vi "FL_SG_Filter_2.vi"(2 "SG coefficients":T1, 3 "Point of interest (can be used for extrapolation)":i32, 4 "Input array of data":dbl[](array[numeric])) -> (1 "Filtered data, 0 order":dbl)   [LabVIEW 2016]
doc: "This VI makes a Savitzky-Golay filtered of input data, length of the fitler is 31 sample, 3rd order polynom. First (and possibly last, depend on filter work mode) 15 values entered into filter will be filtered via simplified Klaman with K=0.3 instead."
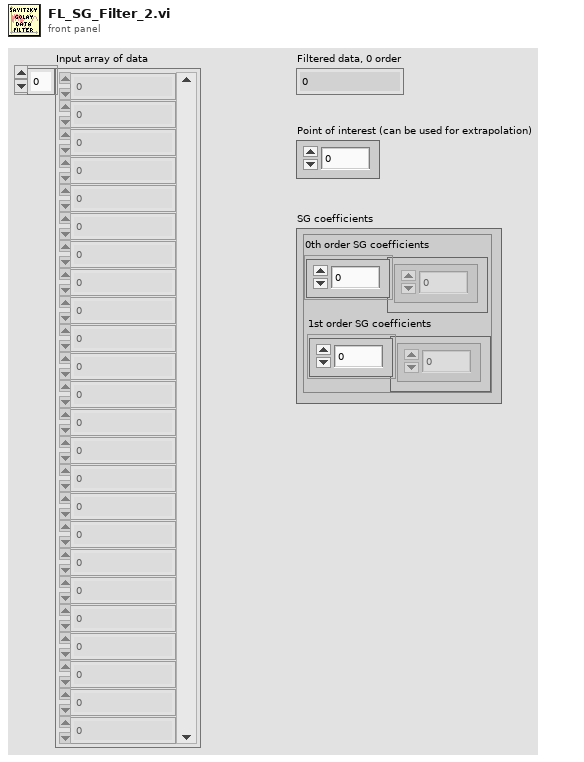
[diagram p1: front panel]
types:
  T1 = cluster{"0th order SG coefficients":dbl[], "1st order SG coefficients":dbl[]}
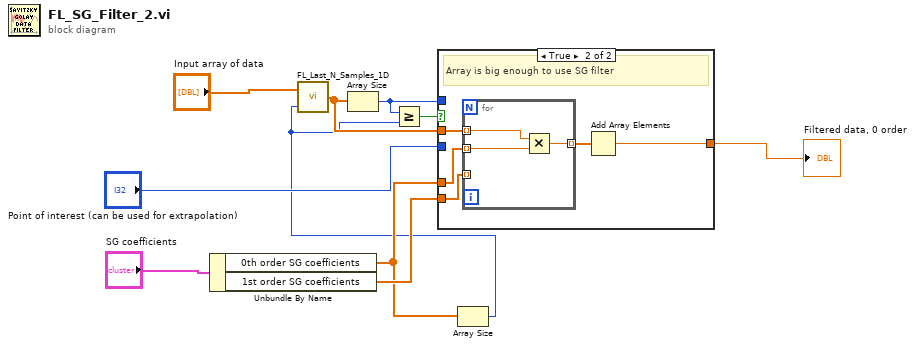
[diagram p0: block diagram]
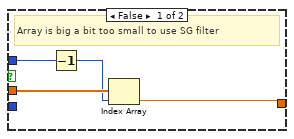
[diagram p2: hidden frame]
diagram:
  n1 = Unbundle By Name("SG coefficients") -> ("0th order SG coefficients"=w2:dbl[], "1st order SG coefficients"=w3:dbl[])
  n2 = Array Size(array=w2) -> (size(s)=w1:i32)
  n3 = call "FL_Last_N_Samples_1D.vi"("BufferLengthSamples"=w1, "Input Array of strings"="Input array of data") -> ("Output Array of strings"=w9:dbl[])
  n4 = Array Size(array=w9) -> (size(s)=w5:i32)
  n5 = Greater Or Equal?(x=w5, y=w1) -> (x >= y?=w8:bool)
  n6 = case shown="True" w8 {
    tunnel: w9 -> [w14 w19]
    tunnel: w2 -> [_ w18]
    tunnel: w3 -> [_ w17]
    tunnel: [w13 w15] -> w7
    tunnel: "Point of interest (can be used for extrapolation)" -> [_ _]
    tunnel: w5 -> [w12 _]
    frame False {
      # "Array is big a bit too small to use SG filter"
      n7 = Decrement(x=w12) -> (x-1=w11:i32)
      n8 = Index Array(array=w14, index=w11) -> (element=w13:dbl)
    }
    frame True {
      # "Array is big enough to use SG filter"
      n9 = for {
        tunnel: w19 -> [w22] mode=indexing
        tunnel: w18 -> [w20] mode=indexing
        tunnel: w17 -> [_] mode=indexing
        tunnel: [w21] -> w16 mode=indexing
        n10 = Multiply(x=w22, y=w20) -> (x*y=w21:dbl)
      }
      n11 = Add Array Elements(numeric array=w16) -> (sum=w15:dbl)
    }
  }
  "Filtered data, 0 order" <- w7
